vi "Read Power Measurement and Step Source.vi"(8 "error in (no error)":errorcluster, 9 "Source Value (0.1)":dbl=0.1, 10 "Source Measure Unit Channel (0: Channel A)":i32(ring) items=["Channel A", "Channel B"], 11 "VISA resource name":refnum<visa-resource-name>) -> (0 "error out":errorcluster, 2 "Power (W)":dbl, 3 "VISA resource name out":refnum<visa-resource-name>)   [LabVIEW 2020, in "Keithley 2600 Series.lvlib"]
doc: "Returns the measured power before stepping the source."
uses:
  <instrlib>/Keithley 2600 Series/Keithley 2600 Series.lvlib
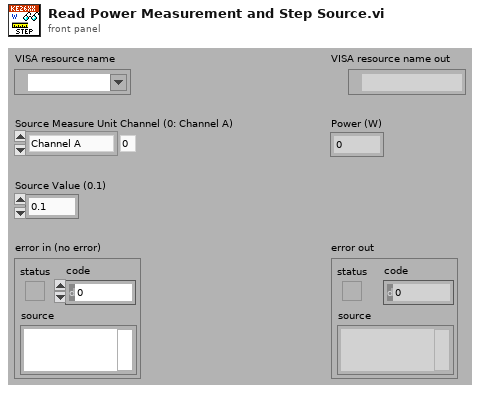
[diagram p1: front panel]
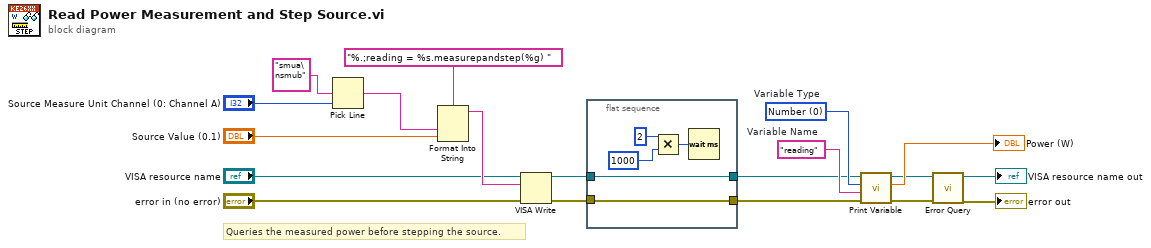
[diagram p0: block diagram]
diagram:
  w6 = "reading"  # Variable Name
  w7 = 0 items=["Number", "Message"]  # Variable Type
  # "Queries the measured power before stepping the source."
  n1 = Pick Line(multi-line string="smua\nsmub", line index="Source Measure Unit Channel (0: Channel A)") -> (output string=w10:string)  [unwired: 1 in]
  n2 = Format Into String(format string="%.;reading = %s.measurepandstep(%g) ", w10, "Source Value (0.1)") -> (resulting string=w17:string)  [unwired: 2 in, 1 out]
  n3 = VISA Write(VISA resource name="VISA resource name", write buffer=w17, error in (no error)="error in (no error)") -> (VISA resource name out=w9:refnum<visa-resource-name>, error out=w8:errorcluster)  [unwired: 1 out]
  n4 = flat-sequence {
    tunnel: w9 -> [w24]
    tunnel: w8 -> [w23]
    tunnel: [w24] -> w5
    tunnel: [w23] -> w4
    frame #0 {
      n5 = Multiply(x=2, y=1000) -> (x*y=w22:i32)
      n6 = Wait (ms)(milliseconds to wait=w22) -> ()  [unwired: 1 out]
    }
  }
  n7 = call <instrlib>:"Print Variable.vi"("error in (no error)"=w4, "Variable Name"=w6, "Variable Type (0: Number)"=w7, "VISA resource name"=w5) -> ("error out"=w2:errorcluster, "Number"=→"Power (W)":dbl, "VISA resource name out"=w1:refnum<visa-resource-name>)  [unwired: 4 in, 1 out]
  n8 = call <instrlib>:"Error Query.vi"("error in (no error)"=w2, "VISA resource name"=w1) -> ("error out"=→"error out":errorcluster, "VISA resource name out"=→"VISA resource name out":refnum<visa-resource-name>)  [unwired: 6 in, 2 out]
